vi "SetTemperature.vi"(4 "Approach":i32(ring) items=["FastSettle", "NoOvershoot"], 6 "Rate":dbl=10.0, 7 "Temperature":dbl=300.0, 8 "error in (no error)":errorcluster, 9 "Instrument Ref In":refnum<k24>) -> (0 "SetTemperature Error":i32, 2 "error out":errorcluster, 3 "Instrument Ref Out":refnum<k24>)   [LabVIEW 2016]
uses:
  C:/user/patrick/hg/levylab_inst_ppms2/lvsrc/PPMS2/QDInstrument_LabView/QDInstrument.dll
  QDInstrument.dll
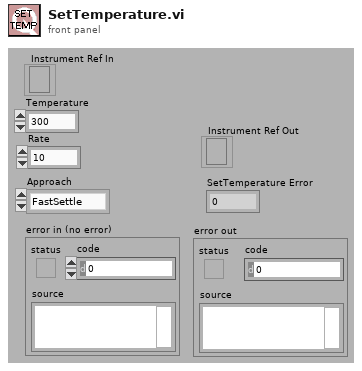
[diagram p1: front panel]
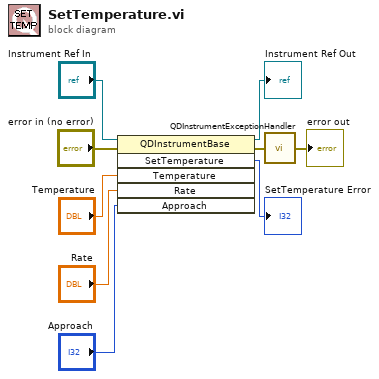
[diagram p0: block diagram]
diagram:
  n1 = invoke class="QDInstrumentBase" method="SetTemperature"(reference="Instrument Ref In", error in="error in (no error)", "Temperature"="Temperature", "Rate"="Rate", "Approach"="Approach") -> (reference out=→"Instrument Ref Out":refnum<k24>, error out=w2:errorcluster, "SetTemperature"=→"SetTemperature Error":i32)  [unwired: 1 in, 3 out]
  n2 = call "QDInstrumentExceptionHandler.vi"("Error in"=w2) -> ("Error out"=→"error out":errorcluster)
